vi "Start Scan (Start to End).vi"(7 "Micropulse # In":i32, 8 "error in (no error)":errorcluster, 9 "Inspection Type":T1 caption="Inspection Type [def: Conventional Tests]", 10 "Scan definition":T2 {"Inspection Resolution" format="%#_6f"; "Scan Start" format="%#_6f"; "Scan Length" format="%#_6f"}, 11 "Axis No.":u8=1) -> (0 "error out":errorcluster, 5 "Micropulse # Out":i32)   [LabVIEW 2026, in "MicroPulse_Driver.lvlib"]
uses:
  MicroPulse_Driver.lvlib
  <instrlib>/Micropulse/Micropulse.lvlib
  Data/Datatypes/MP - MSE Action Condition.ctl
  Data/Datatypes/MP - fly scan range.ctl
  Data/Datatypes/MP - inspection direction.ctl
  Data/Datatypes/MP - fly inspection tests.ctl
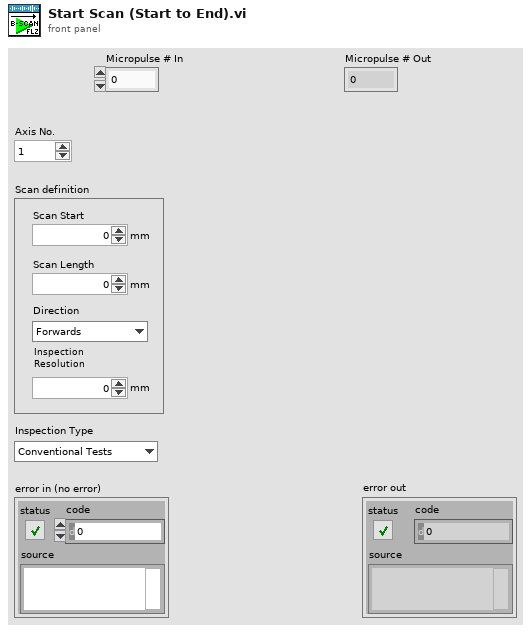
[diagram p1: front panel]
types:
  T1 = typedef "Micropulse.lvlib/MP - fly inspection tests.ctl" = enum16{"Conventional Tests", "Conv >> PA Tests", "PA >> Conv Tests", "PA Tests", "Group Tests", "PA Sweep as per FDEF"}
  T2 = typedef "Micropulse.lvlib/MP - fly scan range.ctl" = cluster{"Scan Start":dbl, "Scan Length":dbl, "Inspection Resolution":dbl, "Direction":T3}
  T3 = typedef "Micropulse.lvlib/MP - inspection direction.ctl" = enum16{"Forwards", "Backwards"}
  T4 = typedef "Micropulse.lvlib/MP - MSE Action Condition.ctl" = enum16{"Normal Stop", "End of FLR or FLZ", "Stall", "Overshoot", "Any Axis Stop"}
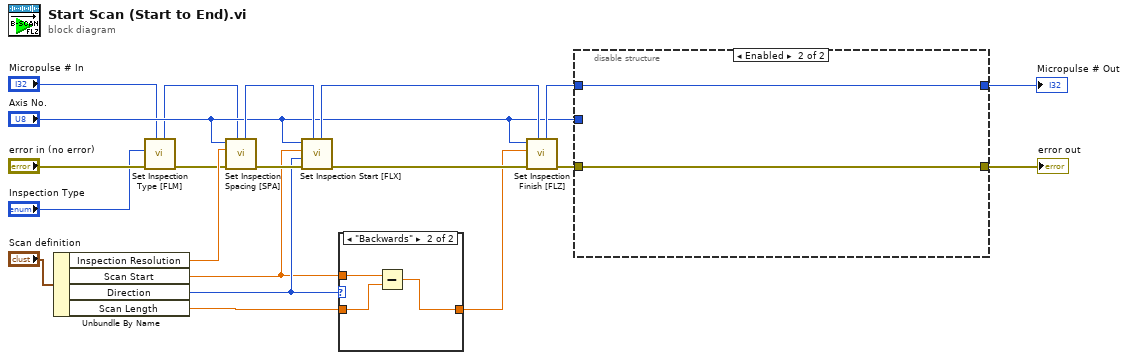
[diagram p0: block diagram]
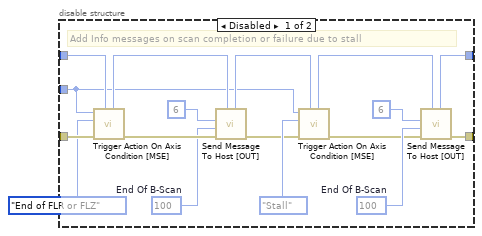
[diagram p2: hidden frame]
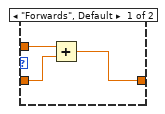
[diagram p3: hidden frame]
diagram:
  n1 = Unbundle By Name("Scan definition") -> ("Inspection Resolution"=w17:dbl, "Scan Start"=w13:dbl, "Direction"=w14:T3, "Scan Length"=w16:dbl)
  n2 = call "Set Inspection Type [FLM].vi"("Micropulse # In"="Micropulse # In", "error in (no error)"="error in (no error)", "Inspection Type"="Inspection Type") -> ("error out"=w4:errorcluster, "Micropulse # Out"=w2:i32)  [unwired: 7 in]
  n3 = call "Set Inspection Spacing [SPA].vi"("Micropulse # In"=w2, "error in (no error)"=w4, "Spacing (mm)"=w17, "Axis No."="Axis No.") -> ("error out"=w19:errorcluster, "Micropulse # Out"=w11:i32)  [unwired: 6 in]
  n4 = call "Set Inspection Start [FLX].vi"("Micropulse # In"=w11, "error in (no error)"=w19, "Direction"=w14, "Start Location (mm)"=w13, "Axis No."="Axis No.") -> ("error out"=w18:errorcluster, "Micropulse # Out"=w10:i32)  [unwired: 5 in]
  n5 = case shown="\"Backwards\"" w14 {
    tunnel: w16 -> [w22 w25]
    tunnel: [w21 w24] -> w15
    tunnel: w13 -> [w23 w26]
    frame "Forwards", Default {
      n6 = Add(x=w23, y=w22) -> (x+y=w21:dbl)
    }
    frame "Backwards" {
      n7 = Subtract(x=w26, y=w25) -> (x-y=w24:dbl)
    }
  }
  n8 = call "Set Inspection Finish [FLZ].vi"("Micropulse # In"=w10, "error in (no error)"=w18, "End Location (mm)"=w15, "Axis No."="Axis No.") -> ("error out"=w12:errorcluster, "Micropulse # Out"=w9:i32)  [unwired: 6 in]
  n9 = disable-structure shown="Enabled" {
    disable-tunnel: w12 -> [w43 w44]
    disable-tunnel: w9 -> [w41 w45]
    disable-tunnel: [w30 w45] -> w8
    disable-tunnel: [w28 w44] -> w7
    disable-tunnel: "Axis No." -> [w27 _]
    frame Disabled {
      w36 = u8 100  # End Of B-Scan
      w37 = u8 100  # End Of B-Scan
      # "Add Info messages on scan completion or failure due to stall"
      n10 = call "Trigger Action On Axis Condition [MSE].vi"("Micropulse # In"=w41, "error in (no error)"=w43, "Action Condition"=MP_-_MSE_Action_Condition."End of FLR or FLZ", "Axis No."=w27) -> ("error out"=w40:errorcluster, "Micropulse # Out"=w39:i32)  [unwired: 6 in]
      n11 = call "Send Message To Host [OUT].vi"("Micropulse # In"=w39, "error in (no error)"=w40, "Parameter"=w37, "Header No."=u8 6) -> ("error out"=w29:errorcluster, "Micropulse # Out"=w31:i32)  [unwired: 6 in]
      n12 = call "Trigger Action On Axis Condition [MSE].vi"("Micropulse # In"=w31, "error in (no error)"=w29, "Action Condition"=MP_-_MSE_Action_Condition."Stall", "Axis No."=w27) -> ("error out"=w33:errorcluster, "Micropulse # Out"=w34:i32)  [unwired: 6 in]
      n13 = call "Send Message To Host [OUT].vi"("Micropulse # In"=w34, "error in (no error)"=w33, "Parameter"=w36, "Header No."=u8 6) -> ("error out"=w28:errorcluster, "Micropulse # Out"=w30:i32)  [unwired: 6 in]
    }
    frame Enabled {
    }
  }
  "error out" <- w7
  "Micropulse # Out" <- w8
